vi "array practice.vi"() -> ()   [LabVIEW 2014]
uses:
  <vilib>/Analysis/Matrix/Datatypes/RealMatrix.ctl
  <vilib>/Analysis/Matrix/NI_Matrix.lvlib
  Control 1.ctl
panel:
  in  "Digital Data":T1
  in  "Array":dbl[](array[numeric])
  in  "Real Matrix":T2
  out "Array 3":dbl[](array[numeric])
  in  "Array 2":dbl[](array[numeric])
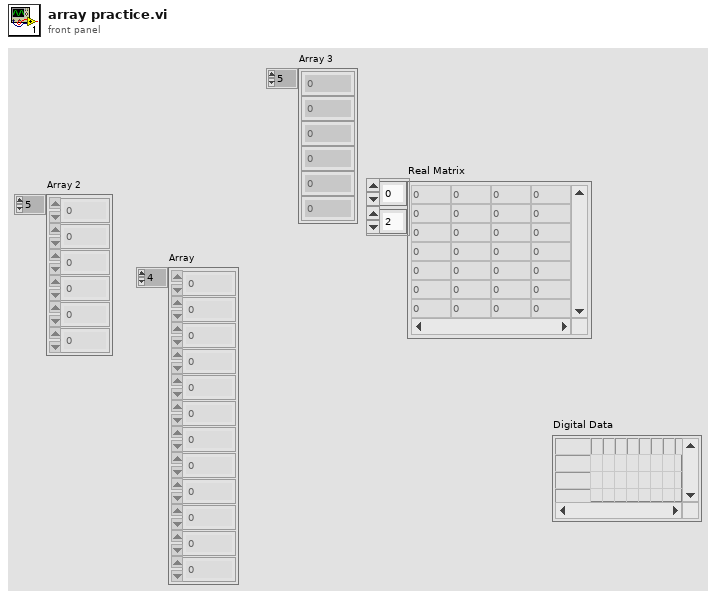
[diagram p1: front panel]
types:
  T1 = typedef "Control 1.ctl" = digitaldata
  T2 = typedef "NI_Matrix.lvlib/RealMatrix.ctl" = dbl[][]
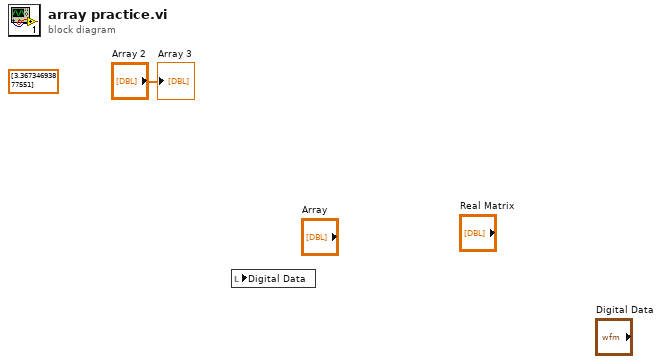
[diagram p0: block diagram]
diagram:
  (unwired) dbl[] [3.36734693877551] ("Array 2")
  n1 = local read "Digital Data"() -> ()  [unwired: 1 in]
  "Array 3" <- "Array 2"
